vi "System Initialization.vi"   [LabVIEW 2020]
uses:
  Globals and TypeDefs/Global Varibal Control.vi
types:
  T1 = typedef "Parameters#2.ctl" = cluster{"MaxBufferSize":i32, "Mag GPIB Address":i32, "Max Current (kA)":dbl, "LTC-GPIB Address":refnum<visa-resource-name>, "Temp Tolerance":dbl}
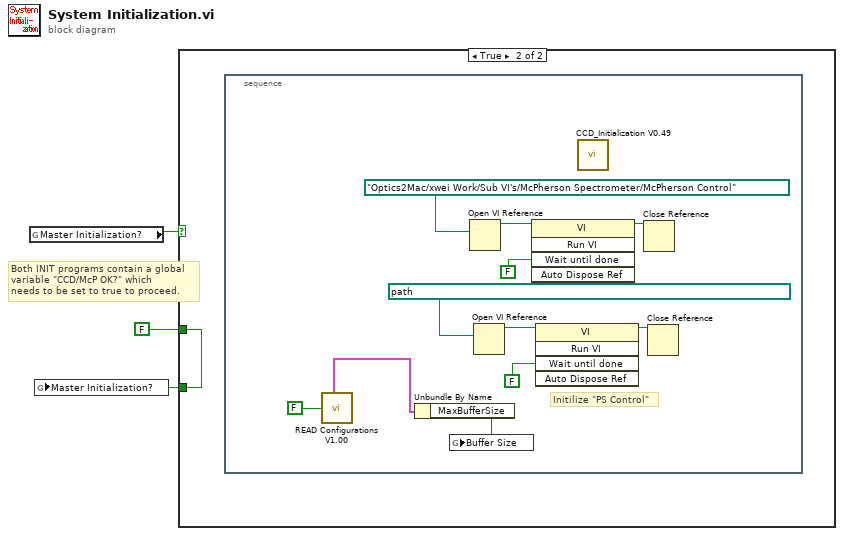
[diagram p0: block diagram]
diagram:
  # "Both INIT programs contain a global\nvariable \"CCD/McP OK?\" which \nneeds to be set to true to proceed."
  n1 = global read "Global Varibal Control.vi" "Master Initialization?"() -> (w3:bool)
  n2 = case shown="True" w3 {
    tunnel: [w4 w5] -> w1
    tunnel: FALSE -> [w4 w5]
    frame False {
    }
    frame True {
      n3 = stacked-sequence {
        frame #0 {
          # "Initilize \"PS Control\""
          n4 = call "READ Configurations V1.00.vi"("OpenParameters(T)orDataBuffers(F)"=FALSE) -> ("Parameters#2"=w7:T1)  [unwired: 2 in, 6 out]
          n5 = Unbundle By Name(w7) -> ("MaxBufferSize"=w8:i32)
          n6 = global write "Global Varibal Control.vi" "Buffer Size"(w8) -> ()
          n7 = Open VI Reference(vi path=path "/Optics2Mac/xwei Work/Sub VI's/McPherson Spectrometer/McPherson Control") -> (vi reference=w10:refnum<vi>)  [unwired: 5 in, 1 out]
          n8 = Open VI Reference(vi path=path "/Optics2Mac/xwei Work/NML Data Acq/Serial Instruments/PS Ä/PS Control") -> (vi reference=w14:refnum<vi>)  [unwired: 5 in, 1 out]
          n9 = invoke class="VI" method="Run VI"(reference=w10, "Wait until done"=FALSE ("Front Panel Window:Open")) -> (reference out=w11:refnum<vi>)  [unwired: 3 in, 4 out]
          n10 = invoke class="VI" method="Run VI"(reference=w14, "Wait until done"=FALSE ("Front Panel Window:Open")) -> (reference out=w15:refnum<vi>)  [unwired: 3 in, 4 out]
          n11 = call "CCD_Initialization V0.49.vi"() -> ()  [unwired: 5 in, 4 out]
          n12 = Close Reference(reference=w11) -> ()  [unwired: 1 in, 1 out]
          n13 = Close Reference(reference=w15) -> ()  [unwired: 1 in, 1 out]
        }
      }
    }
  }
  n14 = global write "Global Varibal Control.vi" "Master Initialization?"(w1) -> ()
